vi "Read Red Tasks.vi"(8 "error in (no error)":errorcluster, 11 "eCRDS in":refnum<class "eCRDS.lvclass">) -> (0 "error out":errorcluster, 2 "Red Tasks":T1={"CLk"="CRDS Red Clk", "AI"="CRDS Red AI", "DO"="CRD Red Laser Output"}, 3 "eCRDS out":refnum<class "eCRDS.lvclass">)   [LabVIEW 2014, in "eCRDS Library.lvlib" / "eCRDS.lvclass"]
uses:
  eCRDS.lvclass
  eCRDS.lvclass/eCRDS.ctl
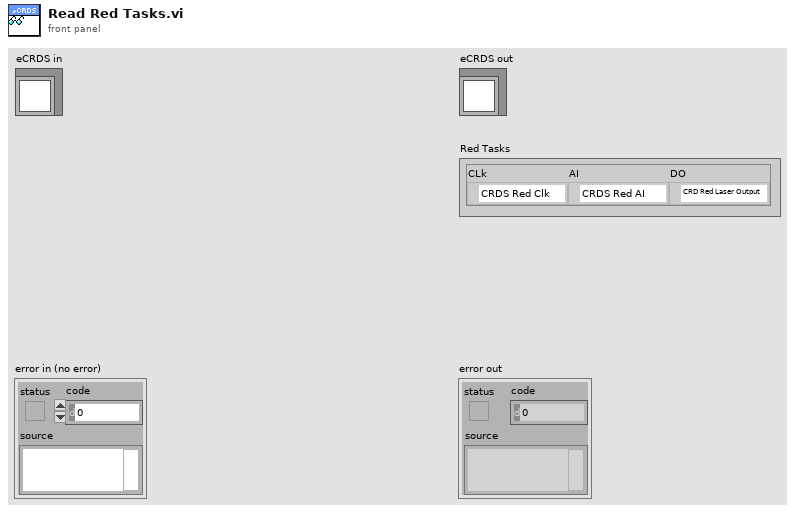
[diagram p1: front panel]
types:
  T1 = cluster{"CLk":refnum<k21>, "AI":refnum<k21>, "DO":refnum<k21>}
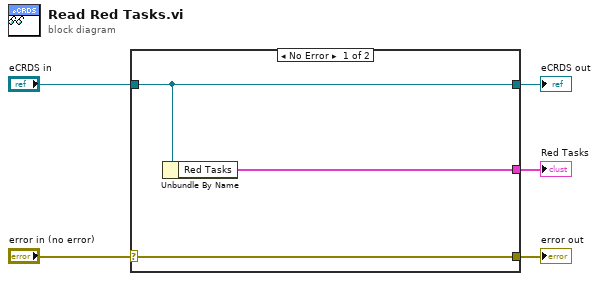
[diagram p0: block diagram]
diagram:
  n1 = case shown="No Error" "error in (no error)" {
    selector: "error in (no error)" -> [w8 w9]
    tunnel: [w8 w9] -> w4
    tunnel: [w7 w10] -> w2
    tunnel: "eCRDS in" -> [w7 w10]
    tunnel: [w6 _] -> w1
    frame No Error {
      n2 = Unbundle By Name(w7) -> ("Red Tasks"=w6:T1)
    }
    frame Error {
    }
  }
  "error out" <- w4
  "eCRDS out" <- w2
  "Red Tasks" <- w1
